vi "led发送数据并接收返回山推.vi"(10 "发送数据":string, 11 "TCP网络连接输入":refnum<k5>) -> (0 "错误输出":errorcluster, 3 "接收到得原始数据":string)   [LabVIEW 2016]
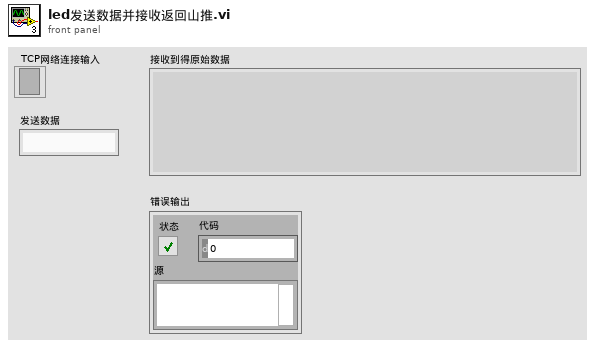
[diagram p1: front panel]
types:
  T1 = enum16{"Standard", "Buffered", "CRLF", "Immediate"}
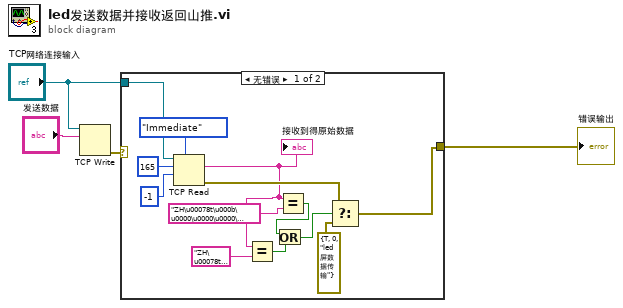
[diagram p0: block diagram]
diagram:
  n1 = TCP Write(connection ID="TCP网络连接输入", data in="发送数据") -> (error out=w1:errorcluster)  [unwired: 2 in, 2 out]
  n2 = case shown="无错误" w1 {
    selector: w1 -> [_ w18]
    tunnel: [w10 w18] -> w2
    tunnel: "TCP网络连接输入" -> [w17 _]
    frame No Error {
      n3 = TCP Read(connection ID=w17, bytes to read=u8 165 ("读取的字节"), 7:T1."Immediate" ("模式（标准）"), 9:-1 ("超时毫秒(25000)")) -> (data out=w8:string, error out=w12:errorcluster)  [unwired: 1 in, 1 out]
      "接收到得原始数据" <- w8
      n4 = Equal?(x=w8, y="ZH\u00078t\u000b\u0000\u0000\u0000\u0000y4\u0001\u0000#\u0000\u0000\u0000\u0000\u0000\u0000\u0000\u0000\u0000\u0000\u0000\u0000.¥") -> (x = y?=w7:bool)
      n5 = Equal?(x=w8, y="ZH\u00078t\u000b\u0000\u0000\u0000\u0000y4\u0001\u0000)D‘\u0000\u0000\u0000\u0000\u0000\u0000\u0000\u0000\u0000\u0000?‰¥") -> (x = y?=w6:bool)
      n6 = Or(x=w6, y=w7) -> (x .or. y?=w5:bool)
      n7 = Select(t=w12, s=w5, f=errorcluster {"status"=TRUE, "code"=0, "source"="led屏数据传输"} ("error IO")) -> (s? t:f=w10:errorcluster)
    }
    frame Error {
    }
  }
  "错误输出" <- w2
